vi "Main.vi"() -> ()   [LabVIEW 2018]
doc: "The myRIO Project template acquires acceleration data from the onboard accelerometer and displays the changes of acceleration values in a waveform chart."
uses:
  <vilib>/Platform/TimedLoop/XDataNode/timing_clust.ctl
  <vilib>/Platform/TimedLoop/XDataNode/nitl_modes.ctl
  <vilib>/Platform/TimedLoop/XDataNode/wakeup.ctl
  <vilib>/myRIO/Instrument Drivers/Onboard IO/DIO/typedefs/DIO Reference.ctl
  <vilib>/myRIO/Common/Instrument Driver Framework/Utilities/typedefs/myRIO Generic Hardware Reference.ctl
  <vilib>/myRIO/Common/Instrument Driver Framework/Utilities/typedefs/Hardware Version Enum.ctl
  <vilib>/myRIO/Common/Instrument Driver Framework/Utilities/typedefs/myRIO v1.0 Reference.ctl
  <vilib>/myRIO/Common/Instrument Driver Framework/Utilities/typedefs/Generic FPGA Reference.ctl
  <vilib>/myRIO/Common/Instrument Driver Framework/myRIO v1.0/DIO/typedefs/DIO Channels List.ctl
  <vilib>/myRIO/Common/Instrument Driver Framework/myRIO v1.0/DIO/typedefs/DIO Channels Enum.ctl
  <vilib>/userdefined/High Color/nirio_resource_hc.ctl
  <vilib>/myRIO/Instrument Drivers/Onboard IO/AI/typedefs/AI Reference.ctl
  <vilib>/myRIO/Common/Instrument Driver Framework/myRIO v1.0/AI/typedefs/AI Channels List.ctl
  <vilib>/myRIO/Common/Instrument Driver Framework/myRIO v1.0/AI/typedefs/AI Channels Enum.ctl
  <vilib>/myRIO/Common/Instrument Driver Framework/Utilities/typedefs/Analog Scaling Constants List.ctl
  <vilib>/myRIO/Common/Instrument Driver Framework/Utilities/typedefs/Analog Scaling Constants.ctl
  <vilib>/myRIO/Instrument Drivers/Onboard IO/AO/typedefs/AO Reference.ctl
  <vilib>/myRIO/Common/Instrument Driver Framework/myRIO v1.0/AO/typedefs/AO Channels List.ctl
  <vilib>/myRIO/Common/Instrument Driver Framework/myRIO v1.0/AO/typedefs/AO Channels Enum.ctl
  <vilib>/myRIO/Common/Instrument Driver Framework/Utilities/vis/Is FPGA Ref Available.vi
  <vilib>/myRIO/Common/Instrument Driver Framework/myRIO v1.0/AI/vis/myRIO v1.1 Open AI.vi
  <vilib>/myRIO/Instrument Drivers/Onboard IO/AI/vis/Read.vi
  <vilib>/myRIO/Common/Instrument Driver Framework/myRIO v1.0/DIO/vis/myRIO v1.1 Open DIO.vi
  <vilib>/myRIO/Instrument Drivers/Onboard IO/DIO/vis/Write.vi
  <vilib>/myRIO/Common/Instrument Driver Framework/myRIO v1.0/AO/vis/myRIO v1.1 Open AO.vi
  <vilib>/myRIO/Instrument Drivers/Onboard IO/AO/vis/Write.vi
  <vilib>/myRIO/Instrument Drivers/Onboard IO/DIO/vis/Read.vi
  <vilib>/myRIO/Common/Instrument Driver Framework/Utilities/vis/Validate Channels.vi
  <vilib>/myRIO/Common/Instrument Driver Framework/myRIO v1.0/AI/vis/myRIO v1.0 Reserve AI.vi
  <vilib>/myRIO/Common/Instrument Driver Framework/myRIO v1.0/DIO/vis/myRIO v1.0 Reserve DIO.vi
  <vilib>/myRIO/Common/Instrument Driver Framework/myRIO v1.0/AO/vis/myRIO v1.0 Reserve AO.vi
  <vilib>/myRIO/Common/Instrument Driver Framework/myRIO v1.0/AI/vis/myRIO v1.0 Build MUX Configuration AI.vi
  <vilib>/myRIO/Common/Instrument Driver Framework/myRIO v1.0/Resource Manager/vis/myRIO v1.0 Reserve Channel List.vi
  <vilib>/myRIO/Common/Instrument Driver Framework/myRIO v1.0/DIO/vis/myRIO v1.0 Build MUX Configuration DIO.vi
  <vilib>/myRIO/Common/Instrument Driver Framework/myRIO v1.0/AO/vis/myRIO v1.0 Build MUX Configuration AO.vi
  <vilib>/myRIO/Common/Instrument Driver Framework/myRIO v1.0/Resource Manager/vis/myRIO v1.0 Reserve Channel.vi
  <vilib>/myRIO/Common/Instrument Driver Framework/myRIO v1.0/Resource Manager/vis/myRIO v1.0 Unreserve Channel.vi
  <vilib>/myRIO/Common/Instrument Driver Framework/myRIO v1.0/Resource Manager/vis/myRIO v1.0 Create Configuration List.vi
  <vilib>/myRIO/Common/Instrument Driver Framework/myRIO v1.0/Resource Manager/vis/myRIO v1.0 Build Mutex Name.vi
  <vilib>/functionblocks/Counter/Pulse Timer/Pulse Timer.vi
  <vilib>/Utility/VariantDataType/GetNumericInfo.vi
  <vilib>/Utility/error.llb/Error Cluster From Error Code.vi
  <vilib>/myRIO/Common/Instrument Driver Framework/myRIO v1.0/myRIO v1.1 Open.vi
  <vilib>/myRIO/Common/Instrument Driver Framework/myRIO v1.0/AI/vis/myRIO v1.0 Get Scaling Constants AI.vi
  <vilib>/myRIO/Common/Instrument Driver Framework/Utilities/vis/IO Manager.vi
  <vilib>/myRIO/Common/Instrument Driver Framework/Utilities/vis/Configuration Manager.vi
  <vilib>/myRIO/Common/Instrument Driver Framework/myRIO v1.0/myRIO v1.0 Close.vi
  <vilib>/myRIO/Common/Instrument Driver Framework/myRIO v1.0/AI/vis/myRIO v1.0 Read AI.vi
  <vilib>/myRIO/Common/Instrument Driver Framework/myRIO v1.0/Resource Manager/vis/myRIO v1.0 Configure IO.vi
  <vilib>/myRIO/Common/Instrument Driver Framework/myRIO v1.0/DIO/vis/myRIO v1.0 Write DIO.vi
  <vilib>/myRIO/Common/Instrument Driver Framework/myRIO v1.0/DIO/vis/myRIO v1.0 Read DIO.vi
  <vilib>/functionblocks/Bistables/SR Bistable/SR Bistable.vi
  <vilib>/myRIO/Common/Instrument Driver Framework/myRIO v1.0/AO/vis/myRIO v1.0 Get Scaling Constants AO.vi
  <vilib>/myRIO/Common/Instrument Driver Framework/myRIO v1.0/AO/vis/myRIO v1.0 Write AO.vi
  <vilib>/Utility/file.llb/Write Delimited Spreadsheet (string).vi
  <vilib>/Platform/TimedLoop/XDataNode/XDataNode.xnode
  <vilib>/functionblocks/FB Core/FB Core.xnode
  <vilib>/myRIO/Express VI/Onboard IO/AI/AI Express VI.xnode
  <vilib>/myRIO/Instrument Drivers/Onboard IO/AI/vis/myRIO AI Open.xnode
  <vilib>/myRIO/Express VI/Onboard IO/DO/DO Express VI.xnode
  <vilib>/myRIO/Instrument Drivers/Onboard IO/DIO/vis/myRIO DIO Open.xnode
  <vilib>/myRIO/Express VI/Onboard IO/DI/DI Express VI.xnode
  <vilib>/myRIO/Express VI/Onboard IO/AO/AO Express VI.xnode
  <vilib>/myRIO/Instrument Drivers/Onboard IO/AO/vis/myRIO AO Open.xnode
  <vilib>/myRIO/Express VI/Onboard Devices/LED/LED Express VI.xnode
  <vilib>/myRIO/Instrument Drivers/Onboard IO/DIO/DIO.lvlib
  <vilib>/myRIO/Instrument Drivers/Onboard IO/AI/AI.lvlib
  <vilib>/myRIO/Instrument Drivers/Onboard IO/AO/AO.lvlib
  <vilib>/functionblocks/NI_FunctionBlock Libraries.lvlib
  <vilib>/Platform/TimedLoop/XDataNode/XDNodeRunTimeDep.lvlib
panel:
  in  "Pump Test":bool
  out "APPS fault":bool
  out "APPS Output (V)":dbl
  out "APPS output %":dbl
  out "Accelaration":dbl(knob) scale=0.0..100.0
  out "APPS pedal travel %":dbl
  out "APPS2 (V) Input (B/AI1 (Pin 5)) 2":dbl
  out "APPS1":dbl(knob) scale=0.0..100.0
  out "APPS2":dbl(knob) scale=0.0..100.0
  out "APPS2 % 2":dbl
  out "APPS1 (V) Input (B/AI1 (Pin 5)) 2":dbl
  out "APPS1 % 2":dbl
  out "Pump out":bool
  out "RTD Status LED":bool
  out "RFE Indicator":bool
  out "AIR + Boolean":bool
  out "AIR +(A9)":dbl
  out "RTD Button":bool
  out "RTD Brake":bool
  out "EN Indicator":bool
  out "RTD Buzzer":bool
  in  "Buzzer test":bool
  in  "RTD Brake Test":bool
  in  "RFE  Test":bool
  in  "EN Test":bool
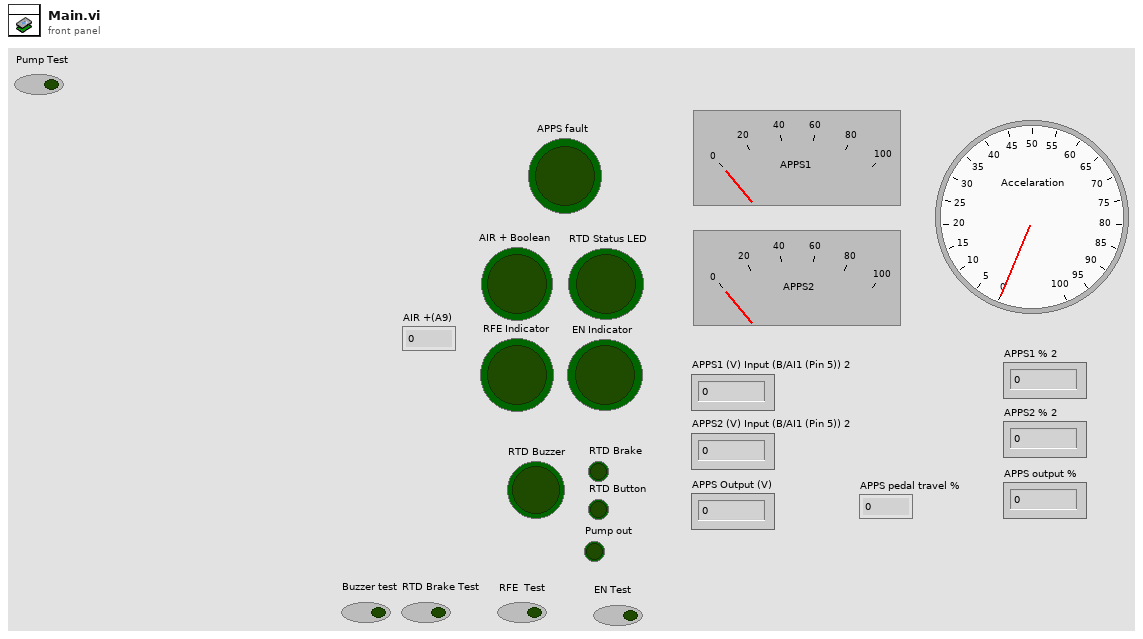
[diagram p1: front panel]
types:
  T1 = typedef "XDNodeRunTimeDep.lvlib/timing_clust.ctl" = cluster{"Expected End [f-1]":u64, "Actual End [f-1]":u64, "Finished Late? [f-1]":bool, "Expected End [i-1]":u64, "Actual End [i-1]":u64, "Finished Late? [i-1]":bool, "Expected Start [i]":u64, "Actual Start [i]":u64, "Expected Start [f]":u64, "Actual Start [f]":u64, "Source Name":string, "Structure Name":string, "Period":i64, "Deadline":i64, "Offset":i64, "Start":i64, "Priority":i32, "Timeout":i32, "Mode":T2, "Wakeup Reason":T3, "Error":errorcluster, "Source Type":string, "Secondary Source Type":string, "Global End Time":u64, "Global Start Time":u64, "Frame Duration":u64, "Iteration Duration":u64, "Assigned CPU":i32, "I/O Scan Engine Mode":u32}
  T2 = typedef "XDNodeRunTimeDep.lvlib/nitl_modes.ctl" = enum32{"No Change", "Process missed periods, maintain original phase", "Discard missed periods, maintain original phase", "Process missed periods, ignore original phase", "Discard missed periods, ignore original phase"}
  T3 = typedef "XDNodeRunTimeDep.lvlib/wakeup.ctl" = enum32{"Normal", "Aborted", "Asynchronous wakeup", "Timing source error", "Timed loop error", "Timeout"}
  T4 = typedef "AI.lvlib/AI Reference.ctl" = cluster{"myRIO Reference":T5, "AI Channels List":T9, "AI Scaling Constants List":T11}
  T5 = typedef "myRIO Generic Hardware Reference.ctl" = cluster{"myRIO Model":T6, "myRIO Hardware Reference":T7}
  T6 = typedef "Hardware Version Enum.ctl" = enum16{"Unknown", "myRIO-1900", "myRIO-1950", "roboRIO", "NI ELVIS RIO CM", "ELVIS III"}
  T7 = typedef "myRIO v1.0 Reference.ctl" = cluster{"Generic FPGA Reference":T8, "Allow multiple opens":bool}
  T8 = typedef "Generic FPGA Reference.ctl" = refnum<k20>
  T9 = typedef "AI Channels List.ctl" = T10[]
  T10 = typedef "AI Channels Enum.ctl" = enum16{"Not Connected", "AudioIn/Left", "AudioIn/Right", "C/AI0", "C/AI1", "A/AI0", "A/AI1", "A/AI2", "A/AI3", "A/AI4", "A/AI5", "A/AI6", "A/AI7", "B/AI0", "B/AI1", "B/AI2", "B/AI3", "B/AI4", "B/AI5", "B/AI6", "B/AI7", "AI/AI0", "AI/AI1", "AI/AI2", "AI/AI3", "A/AI0 (DIFF)", "A/AI1 (DIFF)", "A/AI2 (DIFF)", "A/AI3 (DIFF)", "B/AI0 (DIFF)", "B/AI1 (DIFF)", "B/AI2 (DIFF)", "B/AI3 (DIFF)"}
  T11 = typedef "Analog Scaling Constants List.ctl" = T12[]
  T12 = typedef "Analog Scaling Constants.ctl" = cluster{"LSB Weight (Volts)":dbl, "Offset (Volts)":dbl, "Signed?":bool}
  T13 = typedef "nirio_resource_hc.ctl" = tag
  T14 = typedef "DIO.lvlib/DIO Reference.ctl" = cluster{"myRIO Reference":T5, "DIO Channels List":T15}
  T15 = typedef "DIO Channels List.ctl" = T16[]
  T16 = typedef "DIO Channels Enum.ctl" = enum16{"Not Connected", "C/DIO0", "C/DIO1", "C/DIO2", "C/DIO3", "C/DIO4", "C/DIO5", "C/DIO6", "C/DIO7", "A/DIO0", "A/DIO1", "A/DIO2", "A/DIO3", "A/DIO4", "A/DIO5", "A/DIO6", "A/DIO7", "A/DIO8", "A/DIO9", "A/DIO10", "A/DIO11", "A/DIO12", "A/DIO13", "A/DIO14", "A/DIO15", "A/DIO16", "A/DIO17", "A/DIO18", "A/DIO19", "B/DIO0", "B/DIO1", "B/DIO2", "B/DIO3", "B/DIO4", "B/DIO5", "B/DIO6", "B/DIO7", "B/DIO8", "B/DIO9", "B/DIO10", "B/DIO11", "B/DIO12", "B/DIO13", "B/DIO14", "B/DIO15", "B/DIO16", "B/DIO17", "B/DIO18", "B/DIO19", "LED0", "LED1", "LED2", "LED3", "Button0", "DIO/DIO0", "DIO/DIO1", "DIO/DIO2", "DIO/DIO3", "DIO/DIO4", "DIO/DIO5", "DIO/DIO6", "DIO/DIO7", "DIO/DIO8", "DIO/DIO9", "SPI/CS0", "SPI/CS1", "SPI/CS2", "SPI/CS3", "LED RADIO (Green)", "LED RADIO (Red)", "LED COMM (Green)", "LED COMM (Red)", "LED MODE (Green)", "LED MODE (Red)"}
  T17 = typedef "AO.lvlib/AO Reference.ctl" = cluster{"myRIO Reference":T5, "AO Channel List":T18, "AO Scaling Constant List":T11}
  T18 = typedef "AO Channels List.ctl" = T19[]
  T19 = typedef "AO Channels Enum.ctl" = enum16{"Not Connected", "AudioOut/Left", "AudioOut/Right", "C/AO0", "C/AO1", "A/AO0", "A/AO1", "B/AO0", "B/AO1"}
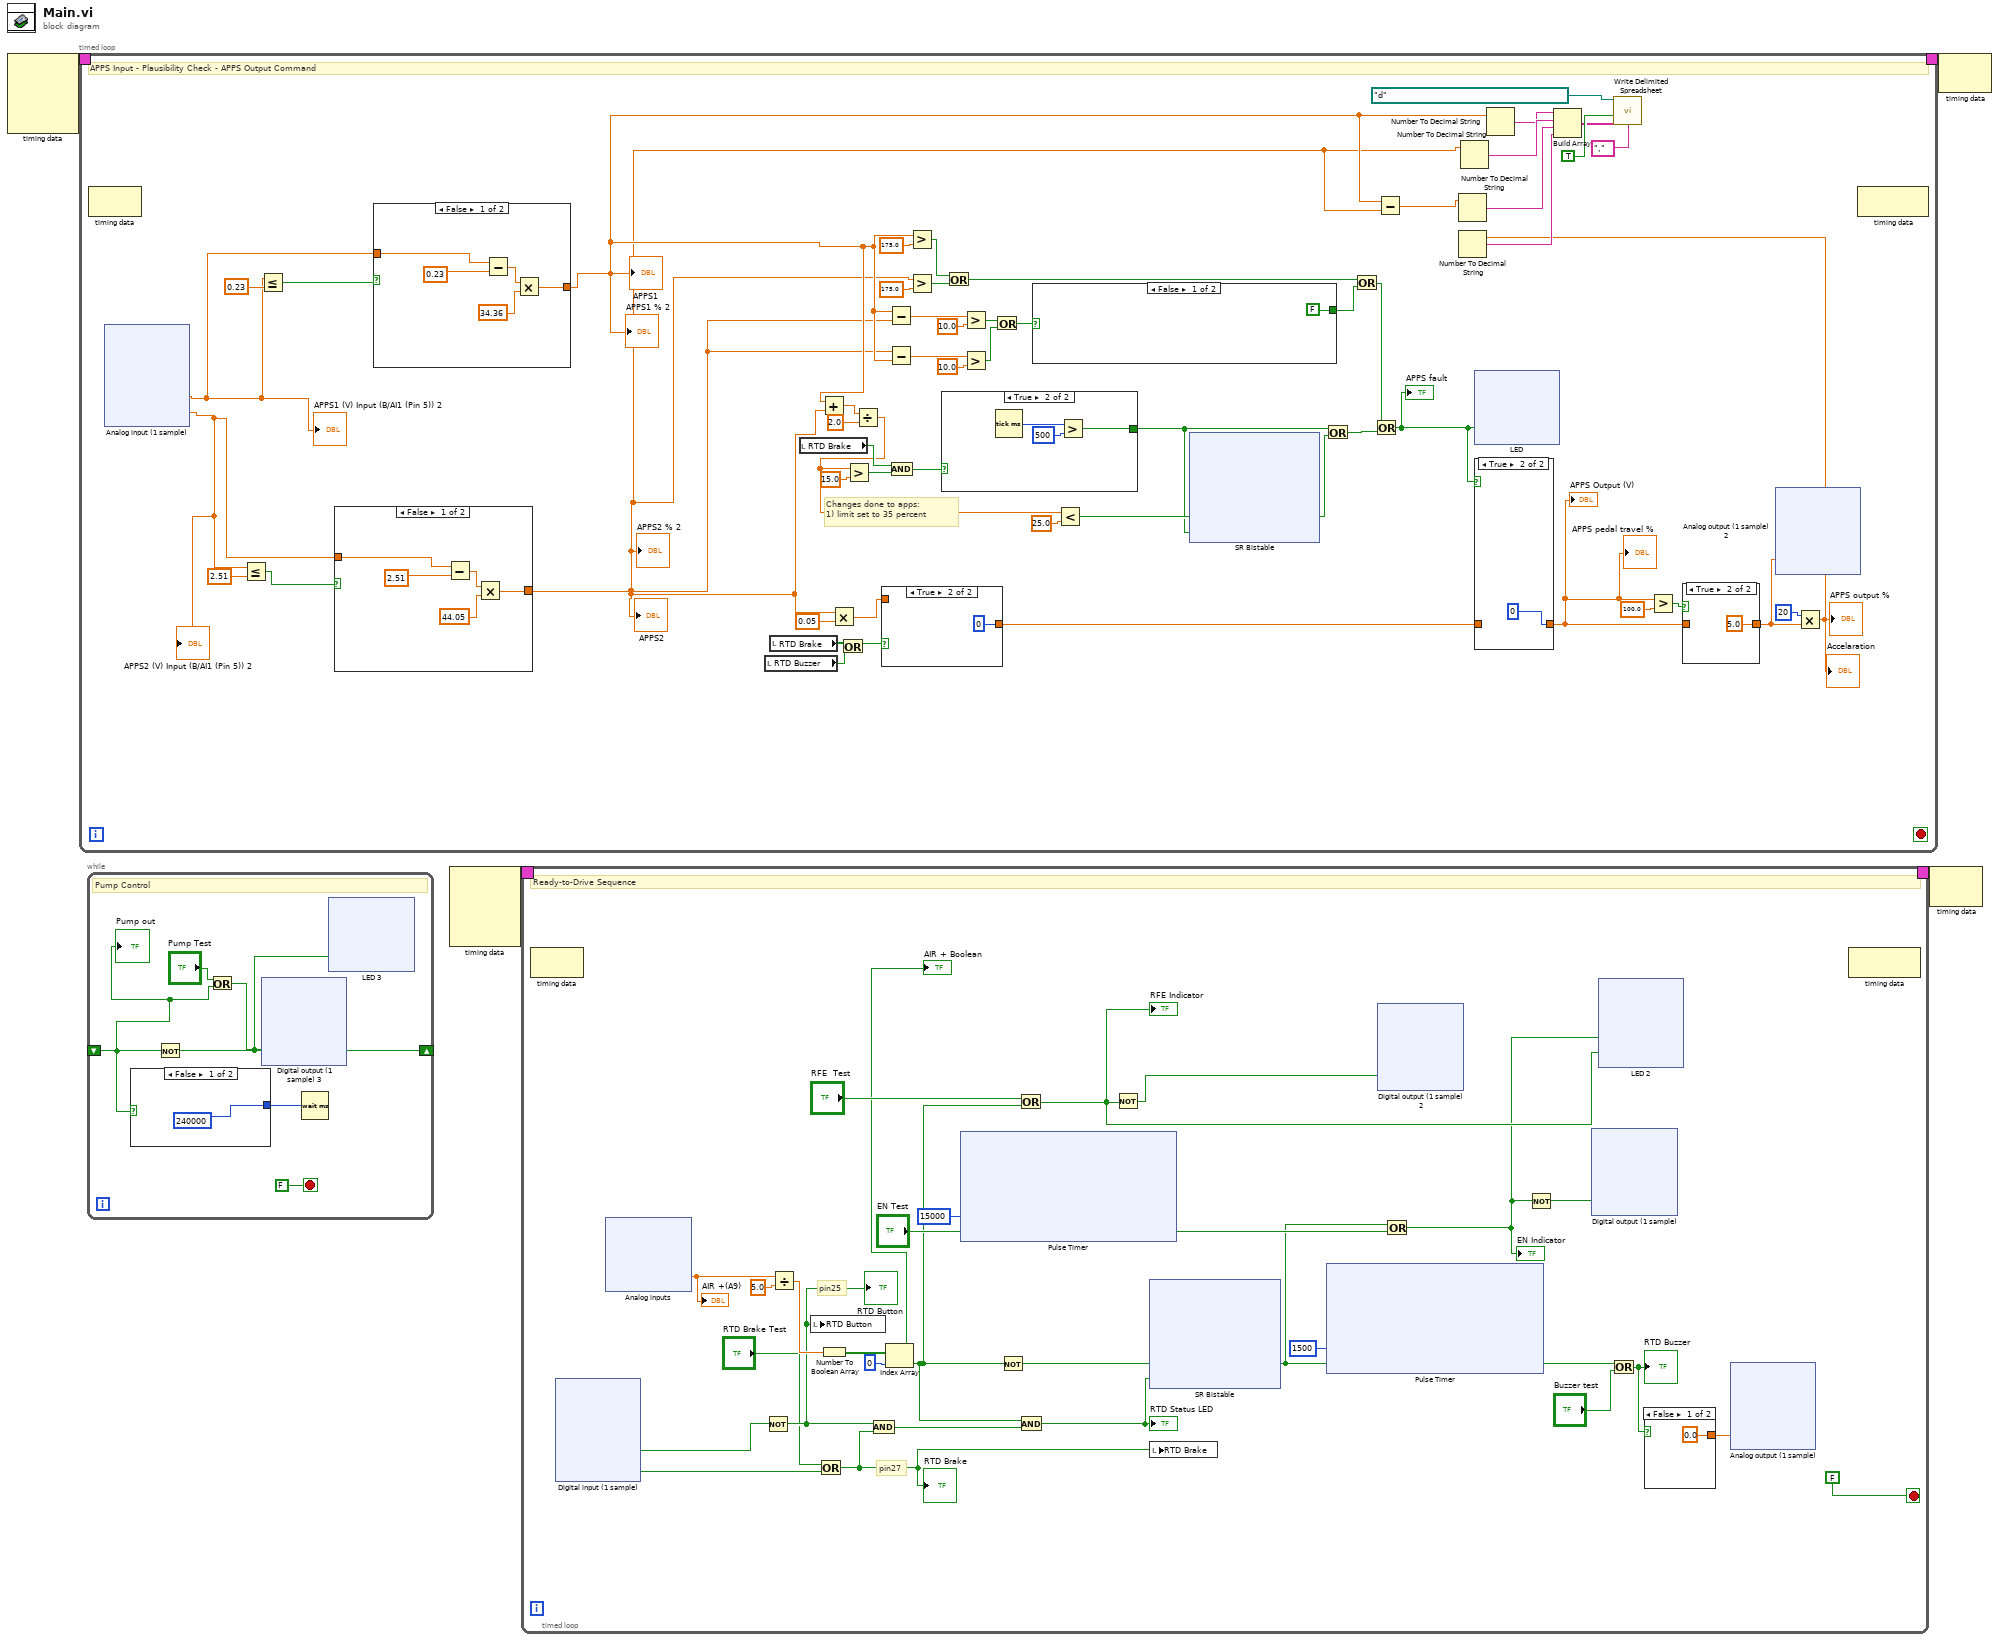
[diagram p0: block diagram]
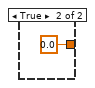
[diagram p2: hidden frame]
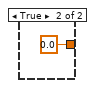
[diagram p3: hidden frame]
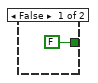
[diagram p4: hidden frame]
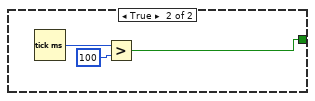
[diagram p5: hidden frame]
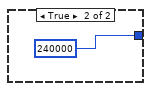
[diagram p9: hidden frame]
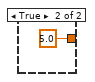
[diagram p10: hidden frame]
diagram:
  n1 = node-c288() -> (w2:T1)  [unwired: 4 in]
  n2 = timed-loop {
    timing: w2 -> [_]
    timing-out: [_] -> w1
    stop <- _ stop-if-true
    # "Changes done to apps:\n1) limit set to 35 percent"
    # "APPS Input - Plausibility Check - APPS Output Command"
    n3 = node-c288() -> ()  [unwired: 1 in, 1 out]
    n4 = xnode "Analog input (1 sample)"() -> ("APPS 1 Input (A/AI2 (Pin 7))"=w7:dbl, "APPS 2 Input (A/AI1 (Pin 5))"=w6:dbl)  [unwired: 1 in, 1 out]
    "APPS2 (V) Input (B/AI1 (Pin 5)) 2" <- w6
    "APPS1 (V) Input (B/AI1 (Pin 5)) 2" <- w7
    n5 = Less Or Equal?(x=w6, y=2.51) -> (x <= y?=w26:bool)
    n6 = Less Or Equal?(x=w7, y=0.23) -> (x <= y?=w24:bool)
    n7 = case shown="False" w26 {
      tunnel: w6 -> [w67 _]
      tunnel: [w66 0.0] -> w12
      frame False {
        n8 = Subtract(x=w67, y=2.51) -> (x-y=w69:dbl)
        n9 = Multiply(x=w69, y=44.05) -> (x*y=w66:dbl)
      }
      frame True {
      }
    }
    "APPS2" <- w12
    "APPS2 % 2" <- w12
    n10 = case shown="False" w24 {
      tunnel: w7 -> [w61 _]
      tunnel: [w60 0.0] -> w13
      frame False {
        n11 = Subtract(x=w61, y=0.23) -> (x-y=w63:dbl)
        n12 = Multiply(x=w63, y=34.36) -> (x*y=w60:dbl)
      }
      frame True {
      }
    }
    "APPS1" <- w13
    "APPS1 % 2" <- w13
    n13 = local read "RTD Buzzer"() -> (w29:bool)
    n14 = local read "RTD Brake"() -> (w23:bool)
    n15 = local read "RTD Brake"() -> (w37:bool)
    n16 = Add(x=w13, y=w12) -> (x+y=w32:dbl)
    n17 = Multiply(x=w12, y=0.05) -> (x*y=w20:dbl)
    n18 = Or(x=w23, y=w29) -> ()  [unwired: 1 out]
    n19 = Divide(x=w32, y=2.0) -> (x/y=w30:dbl)
    n20 = Greater?(x=w30, y=15.0) -> (0:w47:bool)
    n21 = case shown="True" w23 {
      tunnel: [w162 0] -> w44
      tunnel: w20 -> [w162 _]
      frame False {
      }
      frame True {
      }
    }
    n22 = Subtract(x=w13, y=w12) -> (x-y=w57:dbl)
    n23 = Subtract(x=w12, y=w13) -> (x-y=w49:dbl)
    n24 = And(x=w37, y=w47) -> (x .and. y?=w34:bool)
    n25 = Greater?(x=w13, y=175.0) -> (0:w54:bool)
    n26 = Greater?(x=w12, y=175.0) -> (0:w53:bool)
    n27 = case shown="True" w34 {
      tunnel: [FALSE w113] -> w33
      frame False {
      }
      frame True {
        n28 = Tick Count (ms)() -> (millisecond timer value=w115:u32)
        n29 = Greater?(x=w115, y=u32 500) -> (0:w113:bool)
      }
    }
    n30 = Or(x=w54, y=w53) -> (x .or. y?=w52:bool)
    n31 = Greater?(x=w57, y=10.0) -> (0:w58:bool)
    n32 = Greater?(x=w49, y=10.0) -> (0:w50:bool)
    n33 = Or(x=w58, y=w50) -> (x .or. y?=w41:bool)
    n34 = case shown="False" w41 {
      tunnel: [FALSE w159] -> w40
      frame False {
      }
      frame True {
        n35 = Tick Count (ms)() -> (millisecond timer value=w161:u32)
        n36 = Greater?(x=w161, y=u32 100) -> (0:w159:bool)
      }
    }
    n37 = Less?(x=w30, y=25.0) -> (x < y?=w38:bool)
    n38 = xnode "SR Bistable"("reset"=w38, "set"=w33) -> ("output"=w39:bool)  [unwired: 1 in, 1 out]
    n39 = Or(x=w33, y=w39) -> (x .or. y?=w35:bool)
    n40 = Or(x=w52, y=w40) -> (x .or. y?=w36:bool)
    n41 = Or(x=w36, y=w35) -> (x .or. y?=w5:bool)
    "APPS fault" <- w5
    n42 = Subtract(x=w13, y=w12) -> (x-y=w11:dbl)
    n43 = Number To Decimal String(number=w11) -> (decimal integer string=w14:string)  [unwired: 1 in]
    n44 = Number To Decimal String(number=w12) -> (decimal integer string=w19:string)  [unwired: 1 in]
    n45 = xnode "LED"("LED0"=w5) -> ()  [unwired: 1 in, 1 out]
    n46 = case shown="True" w5 {
      tunnel: w44 -> [w166 _]
      tunnel: [w166 0] -> w22
      frame False {
      }
      frame True {
      }
    }
    "APPS Output (V)" <- w22
    "APPS pedal travel %" <- w22
    n47 = Number To Decimal String(number=w13) -> (decimal integer string=w18:string)  [unwired: 1 in]
    n48 = Greater?(x=w22, y=100.0) -> (0:w45:bool)
    n49 = case shown="True" w45 {
      tunnel: [w164 5.0 ("APPS output %")] -> w28
      tunnel: w22 -> [w164 _]
      frame False {
      }
      frame True {
      }
    }
    n50 = xnode "Analog output (1 sample) 2"("APPS Output (B/AO0 (Pin 2))"=w28) -> ()  [unwired: 1 in, 1 out]
    n51 = Multiply(x=20, y=w28) -> (x*y=w9:dbl)
    "APPS output %" <- w9
    "Accelaration" <- w9
    n52 = Number To Decimal String(number=w9) -> (decimal integer string=w10:string)  [unwired: 1 in]
    n53 = Build Array(w18, w19, w14, w10) -> (w8:string[])
    n54 = call-poly <vilib>:"Write Delimited Spreadsheet.vi"("file path (dialog if empty)"=path "d:/", "1D data"=w8, "append to file? (new file:F)"=TRUE, "delimiter (\\t)"="," ("delimiter (\\t)")) -> ()  [unwired: 10 in, 2 out]
    n55 = node-c288() -> ()  [unwired: 1 in, 1 out]
  }
  n56 = while {
    shift-right: [w245] -> _
    shift-left: _ -> [w241]
    stop <- FALSE stop-if-true
    # "Pump Control"
    n57 = case shown="False" w241 {
      tunnel: [240000 240000] -> w244
      frame False {
      }
      frame True {
      }
    }
    n58 = Not(x=w241) -> (.not. x?=w245:bool)
    n59 = Or(x="Pump Test", y=w241) -> (x .or. y?=w240:bool)
    n60 = xnode "Digital output (1 sample) 3"("Pump out (B/DIO7 (Pin 25))"=w240) -> ()  [unwired: 1 in, 1 out]
    n61 = Wait (ms)(milliseconds to wait=w244) -> ()  [unwired: 1 out]
    n62 = xnode "LED 3"("PUMP"=w240) -> ()  [unwired: 1 in, 1 out]
    "Pump out" <- w241
  }
  n63 = node-c288() -> (w4:T1)  [unwired: 4 in]
  n64 = timed-loop {
    timing: w4 -> [_]
    timing-out: [_] -> w3
    stop <- FALSE stop-if-true
    # "pin27"
    # "pin25"
    # "Ready-to-Drive Sequence"
    n65 = node-c288() -> ()  [unwired: 1 in, 1 out]
    n66 = xnode "Digital input (1 sample)"() -> ("RTD Button (B/DIO2 (Pin 15))"=w341:bool, "RTD Brake (B/DIO3 (Pin 17))"=w320:bool)  [unwired: 1 in, 1 out]
    n67 = xnode "Analog inputs"() -> ("AIR + (A/AI3 (Pin 9))"=w324:dbl)  [unwired: 1 in, 1 out]
    "AIR +(A9)" <- w324
    n68 = Not(x=w341) -> (.not. x?=w339:bool)
    "RTD Button" <- w339
    n69 = Divide(x=w324, y=5.0) -> (x/y=w345:dbl)
    n70 = local write "RTD Button"(w339) -> ()
    n71 = Or(x="RTD Brake Test", y=w320) -> (x .or. y?=w336:bool)
    "RTD Brake" <- w336
    n72 = Number To Boolean Array(number=w345) -> (Boolean array=w346:bool[])
    n73 = And(x=w339, y=w336) -> (x .and. y?=w342:bool)
    n74 = Index Array(array=w346, index=0) -> (element=w319:bool)
    "AIR + Boolean" <- w319
    n75 = xnode "Pulse Timer"("preset time (ms)"=15000, "input"="EN Test") -> ("output"=w333:bool)  [unwired: 1 in, 2 out]
    n76 = Not(x=w319) -> (.not. x?=w318:bool)
    n77 = Or(x="RFE  Test", y=w319) -> (x .or. y?=w322:bool)
    "RFE Indicator" <- w322
    n78 = And(x=w319, y=w342) -> (x .and. y?=w338:bool)
    "RTD Status LED" <- w338
    n79 = Not(x=w322) -> (.not. x?=w323:bool)
    n80 = xnode "SR Bistable"("reset"=w318, "set"=w338) -> ("output"=w331:bool)  [unwired: 1 in, 1 out]
    n81 = local write "RTD Brake"(w336) -> ()
    n82 = xnode "Pulse Timer"("preset time (ms)"=1500, "input"=w331) -> ("output"=w329:bool)  [unwired: 1 in, 2 out]
    n83 = xnode "Digital output (1 sample) 2"("RFE (B/DIO0 (Pin 11))"=w323) -> ()  [unwired: 1 in, 1 out]
    n84 = Or(x=w331, y=w333) -> (x .or. y?=w321:bool)
    "EN Indicator" <- w321
    n85 = Not(x=w321) -> (.not. x?=w325:bool)
    n86 = xnode "Digital output (1 sample)"("EN (B/DIO1 (Pin 13))"=w325) -> ()  [unwired: 1 in, 1 out]
    n87 = xnode "LED 2"("EN"=w321, "RFE"=w322) -> ()  [unwired: 1 in, 1 out]
    n88 = Or(x=w329, y="Buzzer test") -> (x .or. y?=w328:bool)
    "RTD Buzzer" <- w328
    n89 = case shown="False" w328 {
      tunnel: [0.0 ("y") 5.0 ("y")] -> w340
      frame False {
      }
      frame True {
      }
    }
    n90 = xnode "Analog output (1 sample)"("RTD - Buzzer (B/AO1 (Pin 4))"=w340) -> ()  [unwired: 1 in, 1 out]
    n91 = node-c288() -> ()  [unwired: 1 in, 1 out]
  }
  n92 = node-c288(w3) -> ()  [unwired: 1 out]
  n93 = node-c288(w1) -> ()  [unwired: 1 out]
